vi "FTW-Message-Compose.vi"(2 "Message Body":string, 3 "Message Header":string, 4 "Sender Identity":string) -> (0 "Message":T1)   [LabVIEW 2013]
uses:
  FTW-Message.ctl
panel:
  # "Inputs"
  # "Outputs"
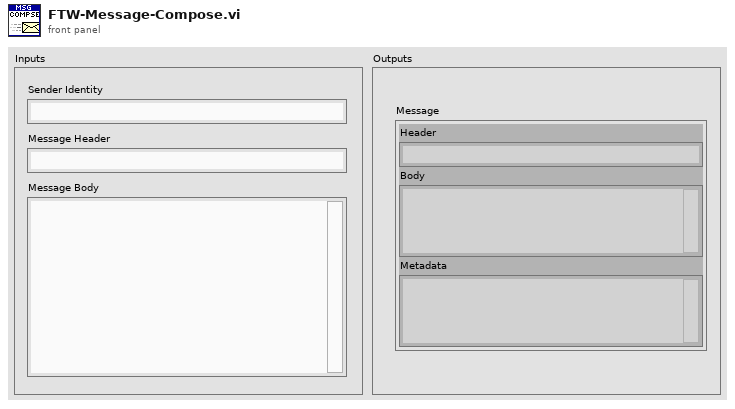
[diagram p1: front panel]
types:
  T1 = typedef "FTW-Message.ctl" = cluster{"Header":string, "Body":string, "Metadata":string}
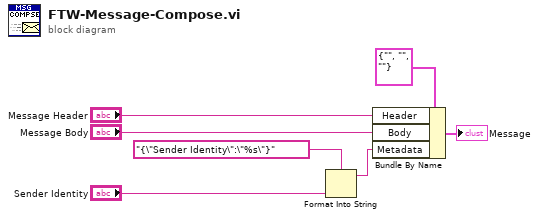
[diagram p0: block diagram]
diagram:
  n1 = Format Into String(format string="{\"Sender Identity\":\"%s\"}", "Sender Identity") -> (resulting string=w2:string)  [unwired: 2 in, 1 out]
  n2 = Bundle By Name(cluster=T1 {"Header"="", "Body"="", "Metadata"=""} ("Message"), "Header"="Message Header", "Body"="Message Body", "Metadata"=w2) -> (→"Message":T1)
